vi "Initiate [TRG].vi"(8 "error in (no error)":errorcluster, 11 "IVI_DCPwr in":refnum<class "IVI_DCPwr.lvclass">) -> (0 "error out":errorcluster, 3 "IVI_DCPwr out":refnum<class "IVI_DCPwr.lvclass">)   [LabVIEW 2013, in "IVI_DCPwr.lvlib" / "IVI_DCPwr.lvclass"]
doc: "This VI initiates output changes that you previously specified. After you call this VI, the power supply waits for the trigger you specify with the IviDCPwr Configure Trigger Source [TRG] VI. After the power supply detects the trigger, it updates its voltage level and current limit to the values you specify with the IviDCPwr Configure Triggered Voltage Level [TRG] and IviDCPwr Configure Triggered Current Limit [TRG] VIs.\n\nNotes:\n\n(1) This VI is part of the IviDCPwrTrigger [TRG] extension group."
uses:
  IVI_DCPwr.lvclass
  IVI_DCPwr.lvclass/IVI_DCPwr.ctl
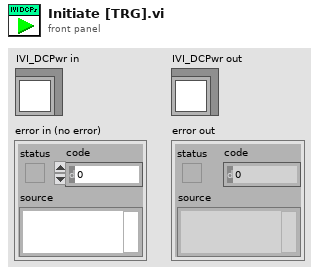
[diagram p1: front panel]
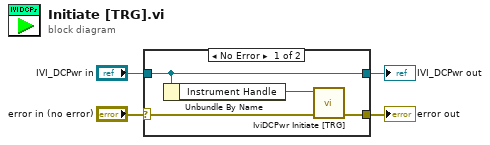
[diagram p0: block diagram]
diagram:
  n1 = case shown="No Error" "error in (no error)" {
    selector: "error in (no error)" -> [w6 w10]
    tunnel: [w5 w10] -> w3
    tunnel: [w8 w9] -> w1
    tunnel: "IVI_DCPwr in" -> [w8 w9]
    frame No Error {
      n2 = Unbundle By Name(w8) -> ("Instrument Handle"=w7:refnum<k15>)
      n3 = call <vilib>:"IviDCPwr Initiate [TRG].vi"("error in (no error)"=w6, "instrument handle"=w7) -> ("error out"=w5:errorcluster)  [unwired: 8 in, 1 out]
    }
    frame Error {
    }
  }
  "error out" <- w3
  "IVI_DCPwr out" <- w1
